vi "Log CAN Frame.vi"(8 "error in (no error)":errorcluster, 9 "timestamp":timestamp, 10 "CAN frame":T1 {"type" items=["CAN Data", "CAN Remote"]; "identifier" format="%.0x"}, 11 "tdms file":refnum<k34>) -> (0 "error out":errorcluster, 3 "tdms file out":refnum<k34>)   [LabVIEW 2014]
uses:
  <vilib>/RioEmbeddedCAN/RioEmbeddedCAN.llb/CANFrameControl.ctl
  MC/MC Temp 1.ctl
  MC/MC Temp 2.ctl
  MC/MC Temp 3.ctl
  MC/MC Position.ctl
  MC/MC Current.ctl
  MC/MC Voltage.ctl
  MC/MC State.ctl
  Inverter States.ctl
  Inverter Run Modes.ctl
  VSM States.ctl
  MC/MC Faults.ctl
  MC/MC Post Faults.ctl
  MC/MC Run Faults.ctl
  MC/MC Torque.ctl
  Global Data.vi
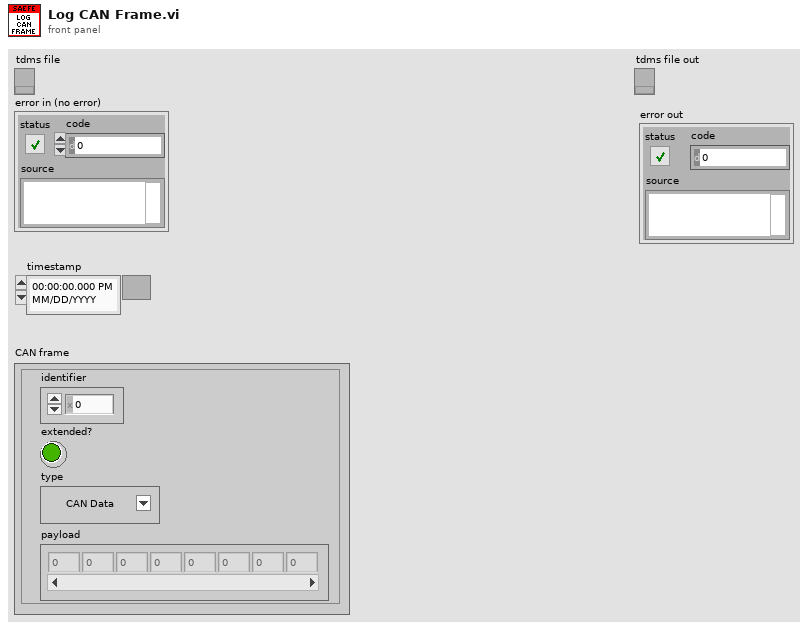
[diagram p1: front panel]
types:
  T1 = typedef "CANFrameControl.ctl" = cluster{"identifier":u32, "extended?":bool, "type":u8, "payload":u8[]}
  T2 = typedef "MC Temp 1.ctl" = cluster{"IGBT A (C)":dbl, "IGBT B (C)":dbl, "IGBT C (C)":dbl, "Gate Driver (C)":dbl}
  T3 = typedef "MC Temp 2.ctl" = cluster{"Control Board (C)":dbl, "RTD #1":dbl, "RTD #2":dbl, "RTD #3":dbl}
  T4 = typedef "MC Temp 3.ctl" = cluster{"RTD #4":dbl, "RTD #5":dbl, "Motor (C)":dbl, "T-Shudder":dbl}
  T5 = typedef "MC Position.ctl" = cluster{"Motor Angle":dbl, "Motor Speed":dbl, "Electrical Output Freq.":dbl, "Delta Resolver Filt.":dbl}
  T6 = typedef "MC Current.ctl" = cluster{"I-Phase A":dbl, "I-Phase B":dbl, "I-Phase C":dbl, "I-Battery":dbl}
  T7 = typedef "MC Voltage.ctl" = cluster{"V-Phase AB":dbl, "V-Phase BC":dbl, "V-Output":dbl, "V-Battery":dbl}
  T8 = typedef "MC State.ctl" = cluster{"Inverter":T9, "Inv. Run Mode":T10, "Inv. Command":enum16{"CAN Mode", "VSM Mode"}, "Inv. Enable":enum16{"Inverter Disabled", "Inverter Enabled"}, "Inv. Enable Lock":enum16{"Inverter Locked", "Inverter Unlocked"}, "Direction":enum16{"Forward", "Reverse/Stopped"}, "VSM States":T11, "Relay 1":bool, "Relay 2":bool, "Relay 3":bool, "Relay 4":bool}
  T9 = typedef "Inverter States.ctl" = enum16{"Power On", "Stop", "Open Loop", "Closed Loop", "Wait", "Internal", "Idle Run", "Idle Stop", ""}
  T10 = typedef "Inverter Run Modes.ctl" = enum16{"Torque Mode", "Speed Mode"}
  T11 = typedef "VSM States.ctl" = enum16{"VSM Start", "Pre-Charge Init", "Pre-Charge Active", "Pre-Charge Complete", "VSM Wait", "VSM Ready", "Motor Running", "Blink Fault Code", "Shutdown in Process", "Recycle Power"}
  T12 = typedef "MC Faults.ctl" = cluster{"POST":T13, "RUN":T14}
  T13 = typedef "MC Post Faults.ctl" = enum32{"None"}
  T14 = typedef "MC Run Faults.ctl" = enum32{"None"}
  T15 = typedef "MC Torque.ctl" = cluster{"T-Requested (Telem)":dbl, "T-Feedback":dbl}
  T16 = enum16{"Off", "On, Not Charging", "Charging", "Charging Finished", "Charging Error"}
  T17 = enum16{"Disconnected", "Pre-charging", "Main Charging", "Balancing", "Charging Finished OK", "Charging Error"}
  T18 = typedef "BMS Telemetry.ctl" = cluster{"Ignition":bool, "Charger Mains":bool, "Fast Charge":bool, "Simple Charger Enabled":bool, "Car State":enum16{"Off", "On, Not Charging", "Charging", "Charging Finished", "Charging Error"}, "Charging State":enum16{"Disconnected", "Pre-charging", "Main Charging", "Balancing", "Charging Finished OK", "Charging Error"}, "Charging Stage Duration":u16, "Last Charging Error":enum16{"No Error", "Cell Voltage Too Low", "No Comm from Cells so can't start", "Maximum charging stage duration expired", "No Comm from Cels so can't balande", "Cannot set balancing voltage", "Cell temps too high", "No Comms so can't determine temp", "# of Cells Mismatch", "Cells Overvoltage", "Cell Protection Event occured."}, "Number of Detected Cells":u8, "Under-Voltage":bool, "Over-Voltage":bool, "Overheat":bool, "Leakage":bool, "No Cell Comms":bool, "Low Voltage":bool, "High Temperature":bool, "Min Cell V":dbl, "Max Cell V":dbl, "Mean Cell V":dbl, "Total V":dbl, "Min Cell t":dbl, "Max Cell t":dbl, "Mean Cell t":dbl, "Cell-V's":dbl[], "Cell-t's":dbl[]}
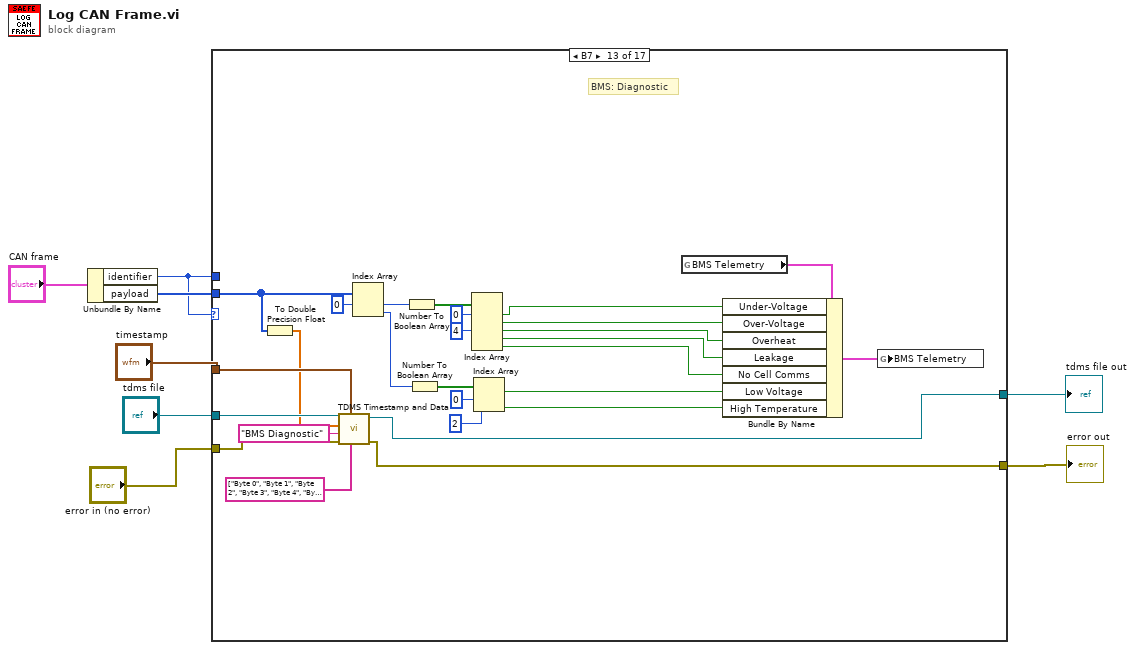
[diagram p0: block diagram]
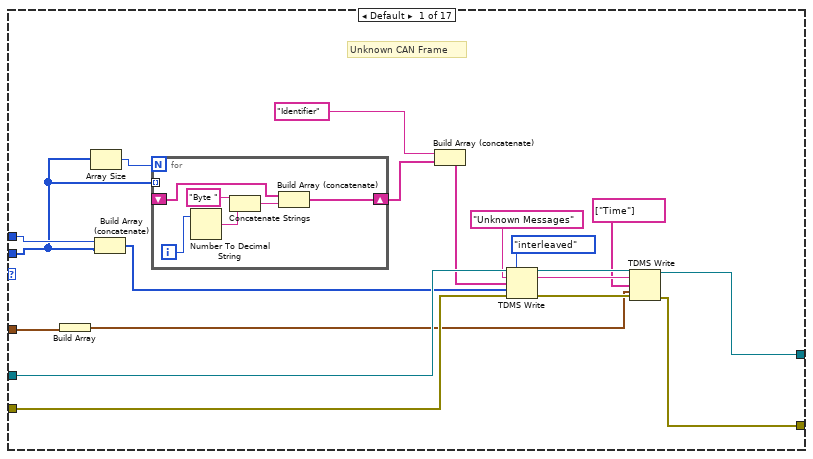
[diagram p2: hidden frame]
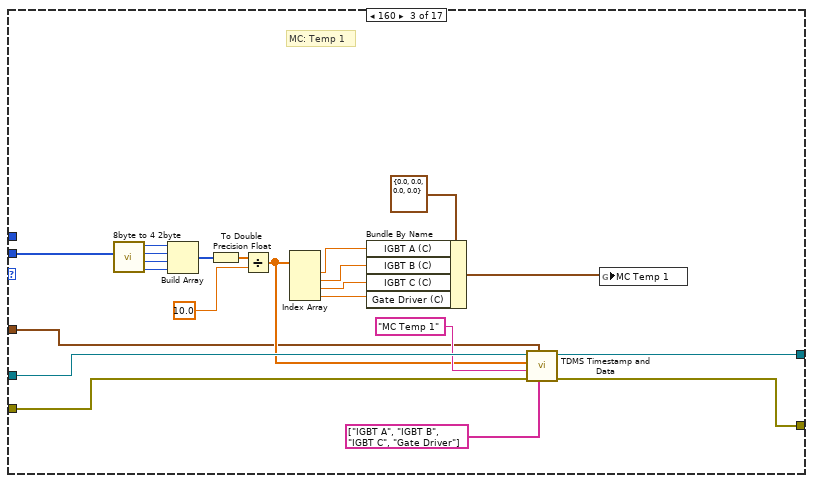
[diagram p4: hidden frame]
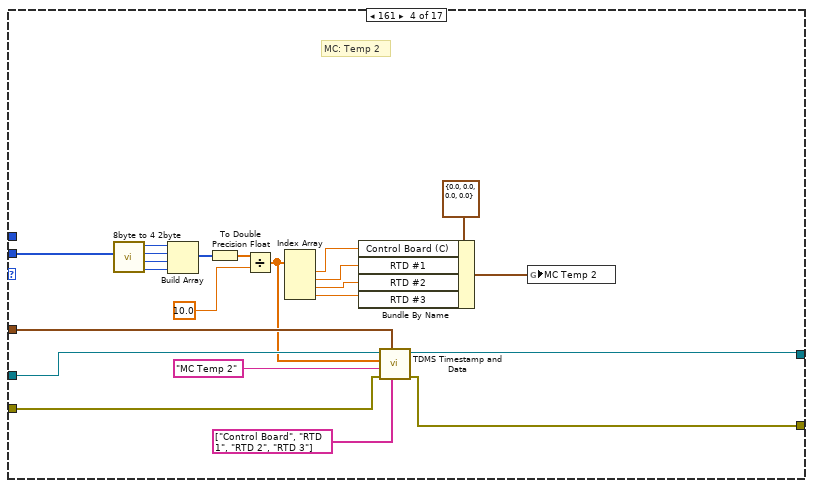
[diagram p5: hidden frame]
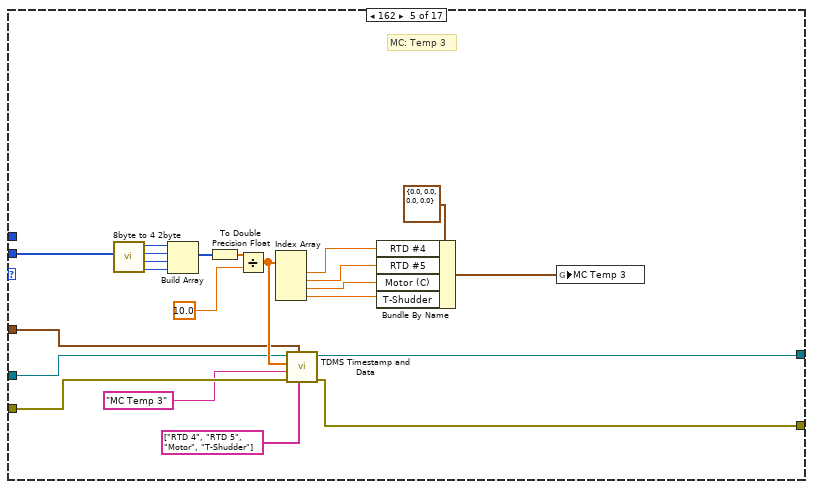
[diagram p6: hidden frame]
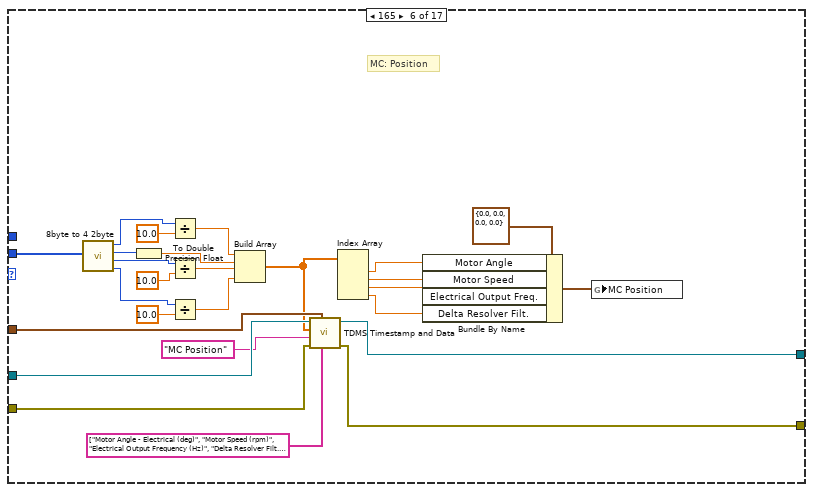
[diagram p7: hidden frame]
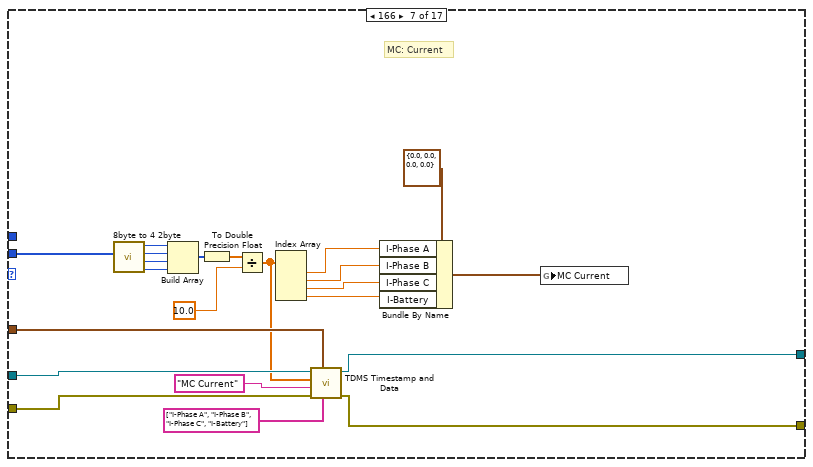
[diagram p8: hidden frame]
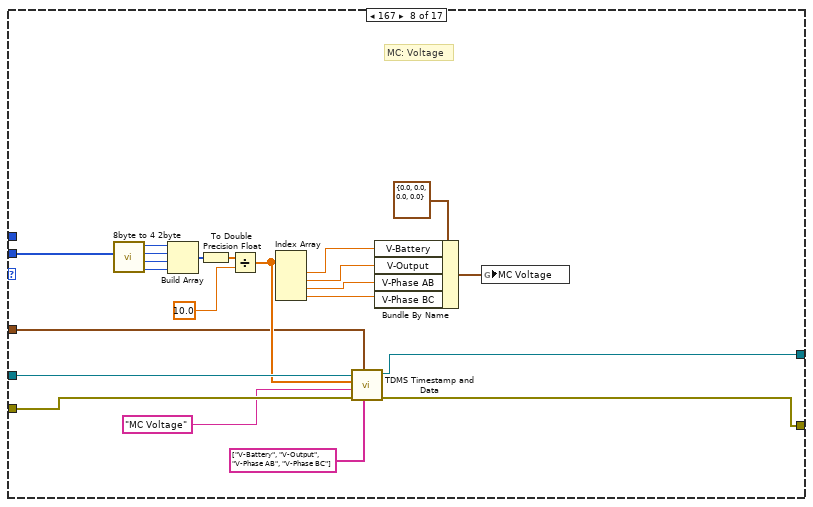
[diagram p9: hidden frame]
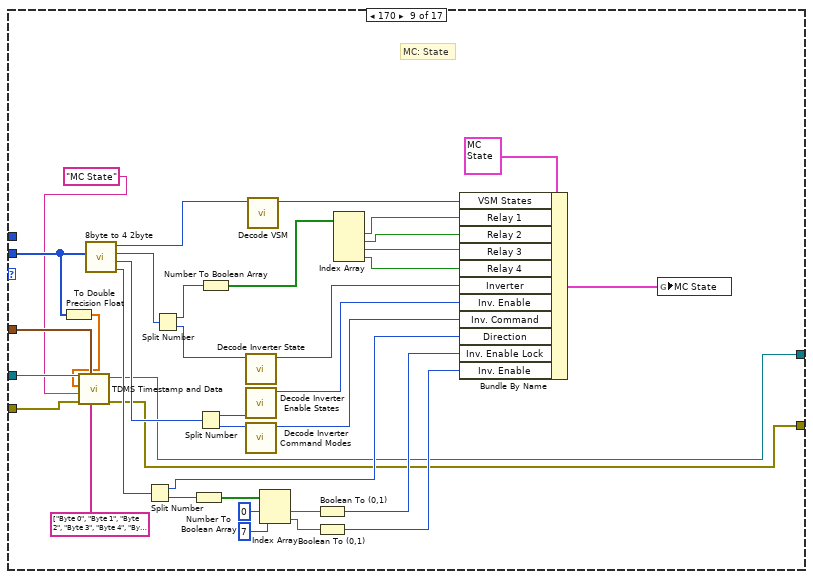
[diagram p10: hidden frame]
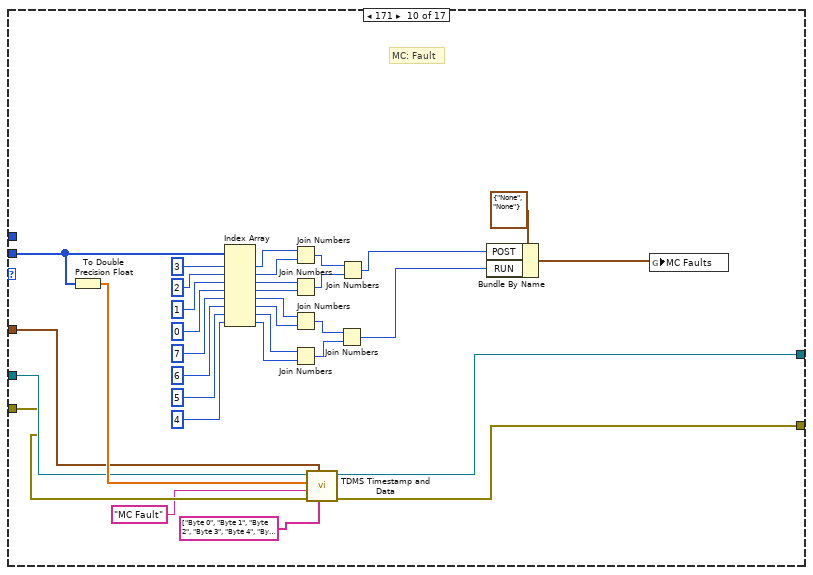
[diagram p11: hidden frame]
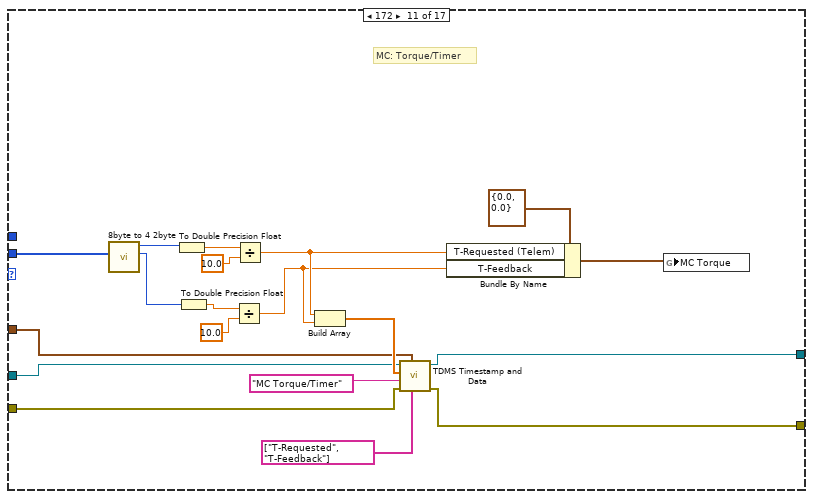
[diagram p12: hidden frame]
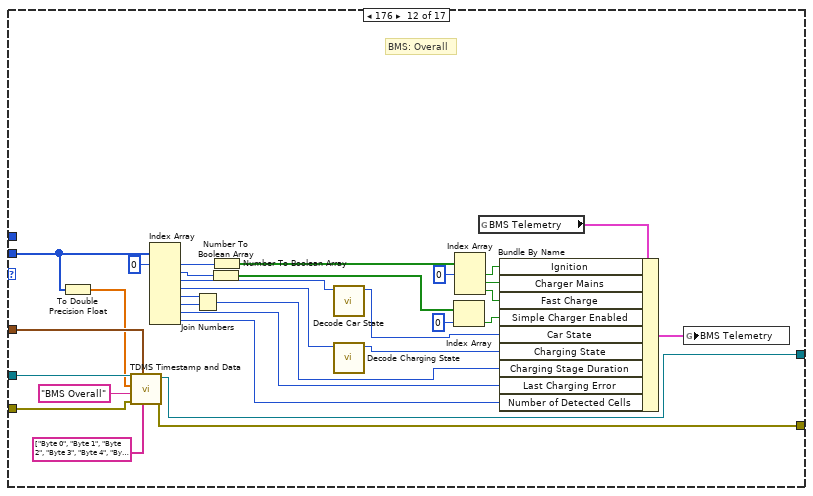
[diagram p13: hidden frame]
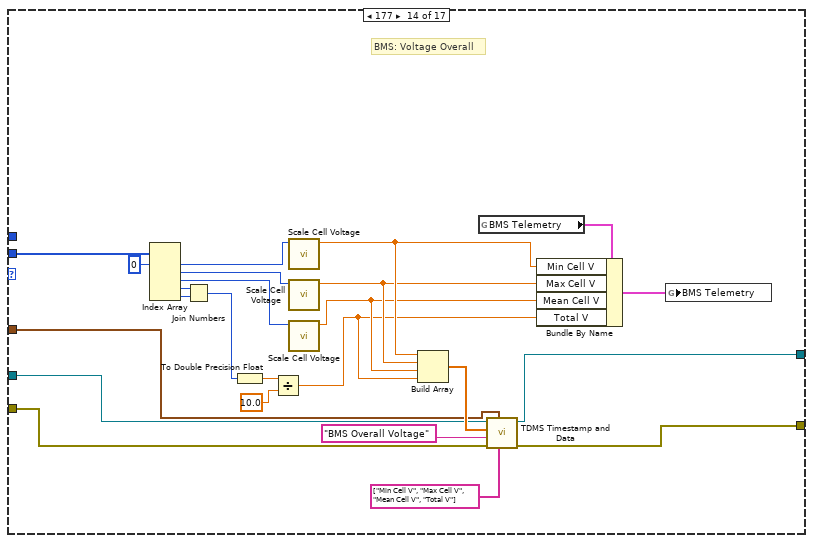
[diagram p14: hidden frame]
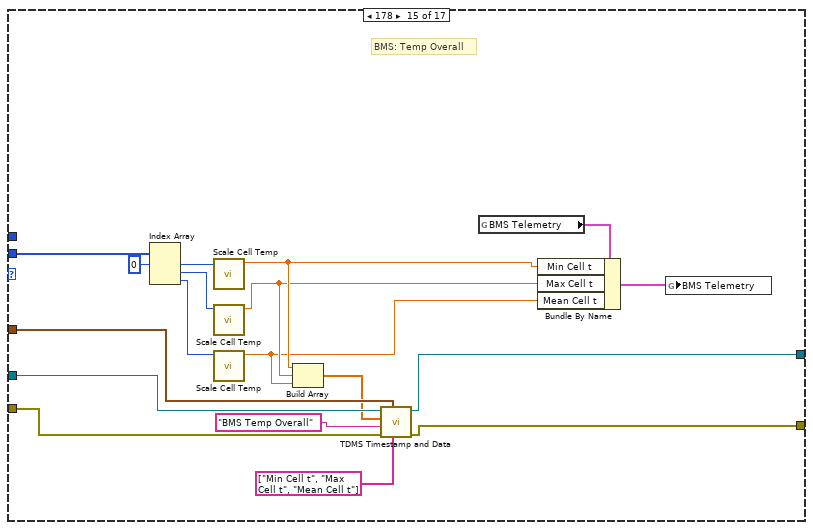
[diagram p15: hidden frame]
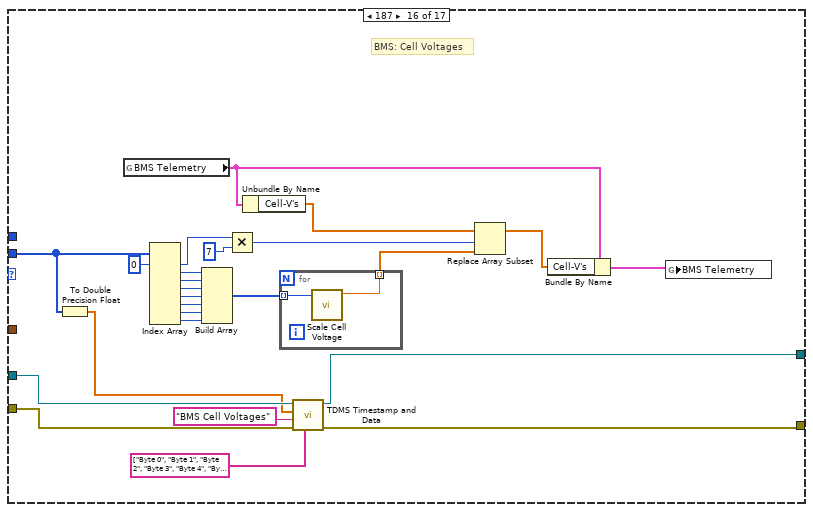
[diagram p16: hidden frame]
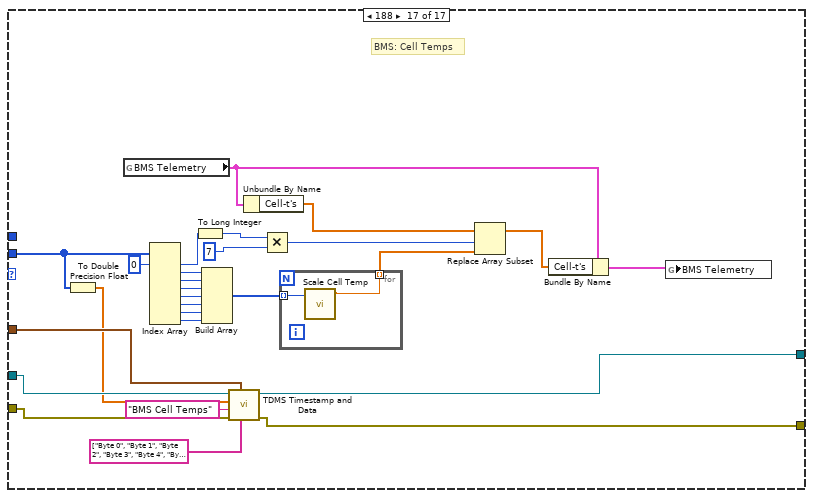
[diagram p17: hidden frame]
diagram:
  n1 = Unbundle By Name("CAN frame") -> ("identifier"=w5:u32, "payload"=w7:u8[])
  n2 = case shown="B7" w5 {
    tunnel: w5 -> [w27 _ _ _ _ _ _ _ _ _ _ _ _ _ _ _ _]
    tunnel: w7 -> [w9 _ w57 w79 w101 w127 w149 w171 w182 w219 w260 w266 w297 w340 w358 w362 w393]
    tunnel: "timestamp" -> [w14 _ w39 w67 w87 w115 w135 w156 w181 w216 w249 w267 w298 w323 w353 _ w398]
    tunnel: "tdms file" -> [w26 w35 w45 w66 w88 w114 w137 w159 w180 w217 w250 w269 w300 w325 w352 w368 w397]
    tunnel: [w11 w35 w42 w63 w85 w111 w131 w154 w177 w213 w246 w263 w294 w321 w344 w365 w394] -> w3
    tunnel: "error in (no error)" -> [w25 w34 w38 w65 w86 w113 w136 w158 w179 w215 w248 w268 w299 w324 w351 w367 w396]
    tunnel: [w12 w34 w41 w64 w84 w112 w130 w153 w176 w212 w245 w262 w293 w320 w343 w364 w395] -> w1
    frame Default {
      # "Unknown CAN Frame"
      n3 = Build Array(w14) -> (w13:timestamp[])
      n4 = Array Size(array=w9) -> (size(s)=w10:i32)
      n5 = Build Array (concatenate)(w27, w9) -> (w24:u32[])
      n6 = for {
        N: w10 -> [_]
        tunnel: w9 -> [_] mode=indexing
        shift-right: [w32] -> w23
        shift-left: _ -> [w28]
        i -> [w31]
        n7 = Number To Decimal String(number=w31) -> (decimal integer string=w30:string)  [unwired: 1 in]
        n8 = Concatenate Strings("Byte " ("string"), w30) -> (w33:string)
        n9 = Build Array (concatenate)(w28, w33) -> (w32:string[])
      }
      n10 = Build Array (concatenate)("Identifier", w23) -> (w21:string[])
      n11 = TDMS Write(0:w26, 1:enum16{"decimated", "interleaved"}."interleaved" ("data layout (0:decimated)"), 5:"Unknown Messages" ("group name in (Untitled)"), 7:w21, 9:w24, 11:w25) -> (4:w18:refnum<k34>, 6:w16:string, 15:w17:errorcluster)  [unwired: 1 out]
      n12 = TDMS Write(0:w18, 5:w16, 7:string[] ["Time"] ("channel name(s) in (Untitled)"), 9:w13, 11:w17) -> (4:w11:refnum<k34>, 15:w12:errorcluster)  [unwired: 1 in, 2 out]
    }
    frame 0 {
      # "Do nothing for NULL frame"
    }
    frame 160 {
      # "MC: Temp 1"
      n13 = call "8byte to 4 2byte.vi"("payload"=w57) -> ("7,6"=w53:i16, "5,4"=w54:i16, "3,2"=w55:i16, "1,0"=w56:i16)  [unwired: 7 in]
      n14 = Build Array(w56, w55, w54, w53) -> (w46:i16[])
      n15 = To Double Precision Float(number=w46) -> (double precision float=w47:dbl[])
      n16 = Divide(x=w47, y=10.0) -> (x/y=w40:dbl[])
      n17 = Index Array(array=w40) -> (element #1=w51:dbl, element #2=w50:dbl, element #3=w49:dbl, element #4=w48:dbl)  [unwired: 4 in]
      n18 = Bundle By Name(cluster=T2 {"IGBT A (C)"=0.0, "IGBT B (C)"=0.0, "IGBT C (C)"=0.0, "Gate Driver (C)"=0.0} ("MC Temp 1"), "IGBT A (C)"=w51, "IGBT B (C)"=w50, "IGBT C (C)"=w49, "Gate Driver (C)"=w48) -> (w36:T2)
      n19 = call "TDMS Timestamp and Data.vi"("channel name(s) in (Untitled)"=string[] ["IGBT A", "IGBT B", "IGBT C", "Gate Driver"], "timestamp"=w39, "error in (no error)"=w38, "group name in (Untitled)"="MC Temp 1", "Array"=w40, "Refnum in"=w45) -> ("error out"=w41:errorcluster, "Refnum out"=w42:refnum<k34>)  [unwired: 4 in]
      n20 = global write "Global Data.vi" "MC Temp 1"(w36) -> ()
    }
    frame 161 {
      # "MC: Temp 2"
      n21 = call "8byte to 4 2byte.vi"("payload"=w79) -> ("7,6"=w75:i16, "5,4"=w76:i16, "3,2"=w77:i16, "1,0"=w78:i16)  [unwired: 7 in]
      n22 = Build Array(w78, w77, w76, w75) -> (w68:i16[])
      n23 = To Double Precision Float(number=w68) -> (double precision float=w69:dbl[])
      n24 = Divide(x=w69, y=10.0) -> (x/y=w62:dbl[])
      n25 = Index Array(array=w62) -> (element #1=w73:dbl, element #2=w72:dbl, element #3=w71:dbl, element #4=w70:dbl)  [unwired: 4 in]
      n26 = Bundle By Name(cluster=T3 {"Control Board (C)"=0.0, "RTD #1"=0.0, "RTD #2"=0.0, "RTD #3"=0.0} ("MC Temp 2"), "Control Board (C)"=w73, "RTD #1"=w72, "RTD #2"=w71, "RTD #3"=w70) -> (w59:T3)
      n27 = call "TDMS Timestamp and Data.vi"("channel name(s) in (Untitled)"=string[] ["Control Board", "RTD 1", "RTD 2", "RTD 3"], "timestamp"=w67, "error in (no error)"=w65, "group name in (Untitled)"="MC Temp 2", "Array"=w62, "Refnum in"=w66) -> ("error out"=w64:errorcluster, "Refnum out"=w63:refnum<k34>)  [unwired: 4 in]
      n28 = global write "Global Data.vi" "MC Temp 2"(w59) -> ()
    }
    frame 162 {
      # "MC: Temp 3"
      n29 = call "8byte to 4 2byte.vi"("payload"=w101) -> ("7,6"=w97:i16, "5,4"=w98:i16, "3,2"=w99:i16, "1,0"=w100:i16)  [unwired: 7 in]
      n30 = Build Array(w100, w99, w98, w97) -> (w90:i16[])
      n31 = To Double Precision Float(number=w90) -> (double precision float=w91:dbl[])
      n32 = Divide(x=w91, y=10.0) -> (x/y=w89:dbl[])
      n33 = Index Array(array=w89) -> (element #1=w95:dbl, element #2=w94:dbl, element #3=w93:dbl, element #4=w92:dbl)  [unwired: 4 in]
      n34 = call "TDMS Timestamp and Data.vi"("channel name(s) in (Untitled)"=string[] ["RTD 4", "RTD 5", "Motor", "T-Shudder"], "timestamp"=w87, "error in (no error)"=w86, "group name in (Untitled)"="MC Temp 3", "Array"=w89, "Refnum in"=w88) -> ("error out"=w84:errorcluster, "Refnum out"=w85:refnum<k34>)  [unwired: 4 in]
      n35 = Bundle By Name(cluster=T4 {"RTD #4"=0.0, "RTD #5"=0.0, "Motor (C)"=0.0, "T-Shudder"=0.0} ("MC Temp 3"), "RTD #4"=w95, "RTD #5"=w94, "Motor (C)"=w93, "T-Shudder"=w92) -> (w81:T4)
      n36 = global write "Global Data.vi" "MC Temp 3"(w81) -> ()
    }
    frame 165 {
      # "MC: Position"
      n37 = call "8byte to 4 2byte.vi"("payload"=w127) -> ("7,6"=w122:i16, "5,4"=w123:i16, "3,2"=w117:i16, "1,0"=w126:i16)  [unwired: 7 in]
      n38 = To Double Precision Float(number=w117) -> (double precision float=w116:dbl)
      n39 = Divide(x=w126, y=10.0) -> (x/y=w121:dbl)
      n40 = Divide(x=w123, y=10.0) -> (x/y=w120:dbl)
      n41 = Divide(x=w122, y=10.0) -> (x/y=w119:dbl)
      n42 = Build Array(w121, w116, w120, w119) -> (w108:dbl[])
      n43 = call "TDMS Timestamp and Data.vi"("channel name(s) in (Untitled)"=string[] ["Motor Angle - Electrical (deg)", "Motor Speed (rpm)", "Electrical Output Frequency (Hz)", "Delta Resolver Filt. (deg)"], "timestamp"=w115, "error in (no error)"=w113, "group name in (Untitled)"="MC Position", "Array"=w108, "Refnum in"=w114) -> ("error out"=w112:errorcluster, "Refnum out"=w111:refnum<k34>)  [unwired: 4 in]
      n44 = Index Array(array=w108) -> (element #1=w107:dbl, element #2=w106:dbl, element #3=w105:dbl, element #4=w104:dbl)  [unwired: 4 in]
      n45 = Bundle By Name(cluster=T5 {"Motor Angle"=0.0, "Motor Speed"=0.0, "Electrical Output Freq."=0.0, "Delta Resolver Filt."=0.0} ("MC Position"), "Motor Angle"=w107, "Motor Speed"=w106, "Electrical Output Freq."=w105, "Delta Resolver Filt."=w104) -> (w102:T5)
      n46 = global write "Global Data.vi" "MC Position"(w102) -> ()
    }
    frame 166 {
      # "MC: Current"
      n47 = call "8byte to 4 2byte.vi"("payload"=w149) -> ("7,6"=w145:i16, "5,4"=w146:i16, "3,2"=w147:i16, "1,0"=w148:i16)  [unwired: 7 in]
      n48 = Build Array(w148, w147, w146, w145) -> (w138:i16[])
      n49 = To Double Precision Float(number=w138) -> (double precision float=w139:dbl[])
      n50 = Divide(x=w139, y=10.0) -> (x/y=w134:dbl[])
      n51 = Index Array(array=w134) -> (element #1=w143:dbl, element #2=w142:dbl, element #3=w141:dbl, element #4=w140:dbl)  [unwired: 4 in]
      n52 = call "TDMS Timestamp and Data.vi"("channel name(s) in (Untitled)"=string[] ["I-Phase A", "I-Phase B", "I-Phase C", "I-Battery"], "timestamp"=w135, "error in (no error)"=w136, "group name in (Untitled)"="MC Current", "Array"=w134, "Refnum in"=w137) -> ("error out"=w130:errorcluster, "Refnum out"=w131:refnum<k34>)  [unwired: 4 in]
      n53 = Bundle By Name(cluster=T6 {"I-Phase A"=0.0, "I-Phase B"=0.0, "I-Phase C"=0.0, "I-Battery"=0.0} ("MC Current"), "I-Phase A"=w143, "I-Phase B"=w142, "I-Phase C"=w141, "I-Battery"=w140) -> (w128:T6)
      n54 = global write "Global Data.vi" "MC Current"(w128) -> ()
    }
    frame 167 {
      # "MC: Voltage"
      n55 = call "8byte to 4 2byte.vi"("payload"=w171) -> ("7,6"=w167:i16, "5,4"=w168:i16, "3,2"=w169:i16, "1,0"=w170:i16)  [unwired: 7 in]
      n56 = Build Array(w170, w169, w168, w167) -> (w160:i16[])
      n57 = To Double Precision Float(number=w160) -> (double precision float=w161:dbl[])
      n58 = Divide(x=w161, y=10.0) -> (x/y=w157:dbl[])
      n59 = Index Array(array=w157) -> (element #1=w165:dbl, element #2=w164:dbl, element #3=w163:dbl, element #4=w162:dbl)  [unwired: 4 in]
      n60 = call "TDMS Timestamp and Data.vi"("channel name(s) in (Untitled)"=string[] ["V-Battery", "V-Output", "V-Phase AB", "V-Phase BC"], "timestamp"=w156, "error in (no error)"=w158, "group name in (Untitled)"="MC Voltage", "Array"=w157, "Refnum in"=w159) -> ("error out"=w153:errorcluster, "Refnum out"=w154:refnum<k34>)  [unwired: 4 in]
      n61 = Bundle By Name(cluster=T7 {"V-Phase AB"=0.0, "V-Phase BC"=0.0, "V-Output"=0.0, "V-Battery"=0.0} ("MC Voltage"), "V-Battery"=w165, "V-Output"=w164, "V-Phase AB"=w163, "V-Phase BC"=w162) -> (w150:T7)
      n62 = global write "Global Data.vi" "MC Voltage"(w150) -> ()
    }
    frame 170 {
      # "MC: State"
      n63 = To Double Precision Float(number=w182) -> (double precision float=w178:dbl[])
      n64 = call "TDMS Timestamp and Data.vi"("channel name(s) in (Untitled)"=string[] ["Byte 0", "Byte 1", "Byte 2", "Byte 3", "Byte 4", "Byte 5", "Byte 6", "Byte 7"], "timestamp"=w181, "error in (no error)"=w179, "group name in (Untitled)"="MC State", "Array"=w178, "Refnum in"=w180) -> ("error out"=w176:errorcluster, "Refnum out"=w177:refnum<k34>)  [unwired: 4 in]
      n65 = call "8byte to 4 2byte.vi"("payload"=w182) -> ("7,6"=w191:i16, "5,4"=w204:i16, "3,2"=w207:i16, "1,0"=w208:i16)  [unwired: 7 in]
      n66 = Split Number(x=w191) -> (hi(x)=w190:u8, lo(x)=w199:u8)
      n67 = Split Number(x=w207) -> (hi(x)=w183:u8, lo(x)=w206:u8)
      n68 = Number To Boolean Array(number=w199) -> (Boolean array=w198:bool[])
      n69 = Split Number(x=w204) -> (hi(x)=w203:u8, lo(x)=w201:u8)
      n70 = Number To Boolean Array(number=w183) -> (Boolean array=w189:bool[])
      n71 = call "Decode Inverter State.vi"("Byte In"=w206) -> ("Inverter State Out"=w205:T9)  [unwired: 10 in]
      n72 = call "Decode Inverter Enable States.vi"("Numeric"=w203) -> ("Inv. Enable"=w202:enum16{"Inverter Disabled", "Inverter Enabled"})  [unwired: 10 in]
      n73 = call "Decode Inverter Command Modes.vi"("Numeric"=w201) -> ("Inv. Command"=w200:enum16{"CAN Mode", "VSM Mode"})  [unwired: 10 in]
      n74 = call "Decode VSM.vi"("VSM Word"=w208) -> ("Enum"=w184:T11)  [unwired: 10 in]
      n75 = Index Array(array=w198, index #1=0 ("index"), index #2=7 ("index")) -> (element #1=w195:bool, element #2=w193:bool)
      n76 = Boolean To (0,1)(Boolean=w195) -> (0, 1=w194:i16)
      n77 = Boolean To (0,1)(Boolean=w193) -> (0, 1=w192:i16)
      n78 = Index Array(array=w189) -> (element #1=w188:bool, element #2=w187:bool, element #3=w186:bool, element #4=w185:bool)  [unwired: 4 in]
      n79 = Bundle By Name(cluster=T8 {"Inverter"=enum."Power On", "Inv. Run Mode"=enum."Torque Mode", "Inv. Command"=enum."CAN Mode", "Inv. Enable"=enum."Inverter Disabled", "Inv. Enable Lock"=enum."Inverter Locked", "Direction"=enum."Forward", "VSM States"=enum."VSM Start", "Relay 1"=FALSE, "Relay 2"=FALSE, "Relay 3"=FALSE, "Relay 4"=FALSE} ("MC State"), "VSM States"=w184, "Relay 1"=w188, "Relay 2"=w187, "Relay 3"=w186, "Relay 4"=w185, "Inverter"=w205, "Inv. Enable"=w202, "Inv. Command"=w200, "Direction"=w190, "Inv. Enable Lock"=w194, "Inv. Enable"=w192) -> (w172:T8)
      n80 = global write "Global Data.vi" "MC State"(w172) -> ()
    }
    frame 171 {
      # "MC: Fault"
      n81 = To Double Precision Float(number=w219) -> (double precision float=w218:dbl[])
      n82 = Index Array(array=w219, index #1=3 ("index"), index #2=2 ("index"), index #3=1 ("index"), index #4=0 ("index"), index #5=7 ("index"), index #6=6 ("index"), index #7=5 ("index"), index #8=4 ("index")) -> (element #1=w229:u8, element #2=w228:u8, element #3=w227:u8, element #4=w226:u8, element #5=w225:u8, element #6=w224:u8, element #7=w223:u8, element #8=w222:u8)
      n83 = Join Numbers(hi=w229, lo=w228) -> ((hi.lo)=w230:u16)
      n84 = Join Numbers(hi=w227, lo=w226) -> ((hi.lo)=w231:u16)
      n85 = Join Numbers(hi=w225, lo=w224) -> ((hi.lo)=w232:u16)
      n86 = Join Numbers(hi=w223, lo=w222) -> ((hi.lo)=w233:u16)
      n87 = call "TDMS Timestamp and Data.vi"("channel name(s) in (Untitled)"=string[] ["Byte 0", "Byte 1", "Byte 2", "Byte 3", "Byte 4", "Byte 5", "Byte 6", "Byte 7"], "timestamp"=w216, "error in (no error)"=w215, "group name in (Untitled)"="MC Fault", "Array"=w218, "Refnum in"=w217) -> ("error out"=w212:errorcluster, "Refnum out"=w213:refnum<k34>)  [unwired: 4 in]
      n88 = Join Numbers(hi=w232, lo=w233) -> ((hi.lo)=w220:u32)
      n89 = Join Numbers(hi=w230, lo=w231) -> ((hi.lo)=w221:u32)
      n90 = Bundle By Name(cluster=T12 {"POST"=enum."None", "RUN"=enum."None"} ("MC Faults"), "POST"=w221, "RUN"=w220) -> (w209:T12)
      n91 = global write "Global Data.vi" "MC Faults"(w209) -> ()
    }
    frame 172 {
      # "MC: Torque/Timer"
      n92 = call "8byte to 4 2byte.vi"("payload"=w260) -> ("3,2"=w256:i16, "1,0"=w259:i16)  [unwired: 7 in, 2 out]
      n93 = To Double Precision Float(number=w259) -> (double precision float=w258:dbl)
      n94 = To Double Precision Float(number=w256) -> (double precision float=w255:dbl)
      n95 = Divide(x=w255, y=10.0) -> (x/y=w252:dbl)
      n96 = Divide(x=w258, y=10.0) -> (x/y=w253:dbl)
      n97 = Build Array(w253, w252) -> (w251:dbl[])
      n98 = call "TDMS Timestamp and Data.vi"("channel name(s) in (Untitled)"=string[] ["T-Requested", "T-Feedback"], "timestamp"=w249, "error in (no error)"=w248, "group name in (Untitled)"="MC Torque/Timer", "Array"=w251, "Refnum in"=w250) -> ("error out"=w245:errorcluster, "Refnum out"=w246:refnum<k34>)  [unwired: 4 in]
      n99 = Bundle By Name(cluster=T15 {"T-Requested (Telem)"=0.0, "T-Feedback"=0.0} ("MC Torque"), "T-Requested (Telem)"=w253, "T-Feedback"=w252) -> (w243:T15)
      n100 = global write "Global Data.vi" "MC Torque"(w243) -> ()
    }
    frame 176 {
      # "BMS: Overall"
      n101 = To Double Precision Float(number=w266) -> (double precision float=w265:dbl[])
      n102 = call "TDMS Timestamp and Data.vi"("channel name(s) in (Untitled)"=string[] ["Byte 0", "Byte 1", "Byte 2", "Byte 3", "Byte 4", "Byte 5", "Byte 6", "Byte 7"], "timestamp"=w267, "error in (no error)"=w268, "group name in (Untitled)"="BMS Overall", "Array"=w265, "Refnum in"=w269) -> ("error out"=w262:errorcluster, "Refnum out"=w263:refnum<k34>)  [unwired: 4 in]
      n103 = Index Array(array=w266, index #1=0 ("index")) -> (element #1=w288:u8, element #2=w282:u8, element #3=w277:u8, element #4=w276:u8, element #5=w274:u8, element #6=w273:u8, element #7=w271:u8, element #8=w270:u8)  [unwired: 7 in]
      n104 = Join Numbers(hi=w274, lo=w273) -> ((hi.lo)=w272:u16)
      n105 = Number To Boolean Array(number=w282) -> (Boolean array=w280:bool[])
      n106 = Number To Boolean Array(number=w288) -> (Boolean array=w287:bool[])
      n107 = call "Decode Car State.vi"("Numeric"=w277) -> ("Car State"=w278:T16)  [unwired: 10 in]
      n108 = call "Decode Charging State.vi"("Numeric"=w276) -> ("Charging State"=w275:T17)  [unwired: 10 in]
      n109 = Index Array(array=w280, index=0) -> (element=w281:bool)
      n110 = Index Array(array=w287, index #1=0 ("index")) -> (element #1=w285:bool, element #2=w284:bool, element #3=w283:bool)  [unwired: 2 in]
      n111 = global read "Global Data.vi" "BMS Telemetry"() -> (w291:T18)
      n112 = Bundle By Name(cluster=w291, "Ignition"=w285, "Charger Mains"=w284, "Fast Charge"=w283, "Simple Charger Enabled"=w281, "Car State"=w278, "Charging State"=w275, "Charging Stage Duration"=w272, "Last Charging Error"=w271, "Number of Detected Cells"=w270) -> (w290:T18)
      n113 = global write "Global Data.vi" "BMS Telemetry"(w290) -> ()
    }
    frame 183 {
      # "BMS: Diagnostic"
      n114 = To Double Precision Float(number=w297) -> (double precision float=w296:dbl[])
      n115 = call "TDMS Timestamp and Data.vi"("channel name(s) in (Untitled)"=string[] ["Byte 0", "Byte 1", "Byte 2", "Byte 3", "Byte 4", "Byte 5", "Byte 6", "Byte 7"], "timestamp"=w298, "error in (no error)"=w299, "group name in (Untitled)"="BMS Diagnostic", "Array"=w296, "Refnum in"=w300) -> ("error out"=w293:errorcluster, "Refnum out"=w294:refnum<k34>)  [unwired: 4 in]
      n116 = Index Array(array=w297, index #1=0 ("index")) -> (element #1=w315:u8, element #2=w306:u8)  [unwired: 1 in]
      n117 = Number To Boolean Array(number=w315) -> (Boolean array=w314:bool[])
      n118 = Number To Boolean Array(number=w306) -> (Boolean array=w305:bool[])
      n119 = Index Array(array=w314, index #1=0 ("index"), index #3=4 ("index")) -> (element #1=w312:bool, element #2=w311:bool, element #3=w309:bool, element #4=w308:bool, element #5=w307:bool)  [unwired: 3 in]
      n120 = Index Array(array=w305, index #1=0 ("index"), index #2=2 ("index")) -> (element #1=w302:bool, element #2=w301:bool)
      n121 = global read "Global Data.vi" "BMS Telemetry"() -> (w318:T18)
      n122 = Bundle By Name(cluster=w318, "Under-Voltage"=w312, "Over-Voltage"=w311, "Overheat"=w309, "Leakage"=w308, "No Cell Comms"=w307, "Low Voltage"=w302, "High Temperature"=w301) -> (w317:T18)
      n123 = global write "Global Data.vi" "BMS Telemetry"(w317) -> ()
    }
    frame 177 {
      # "BMS: Voltage Overall"
      n124 = Index Array(array=w340, index #1=0 ("index")) -> (element #1=w338:u8, element #2=w337:u8, element #3=w336:u8, element #4=w335:u8, element #5=w334:u8)  [unwired: 4 in]
      n125 = Join Numbers(hi=w335, lo=w334) -> ((hi.lo)=w333:u16)
      n126 = To Double Precision Float(number=w333) -> (double precision float=w332:dbl)
      n127 = Divide(x=w332, y=10.0) -> (x/y=w327:dbl)
      n128 = call "Scale Cell Voltage.vi"("Numeric in"=w338) -> ("Numeric out"=w330:dbl)  [unwired: 10 in]
      n129 = call "Scale Cell Voltage.vi"("Numeric in"=w337) -> ("Numeric out"=w329:dbl)  [unwired: 10 in]
      n130 = call "Scale Cell Voltage.vi"("Numeric in"=w336) -> ("Numeric out"=w328:dbl)  [unwired: 10 in]
      n131 = Build Array(w330, w329, w328, w327) -> (w326:dbl[])
      n132 = global read "Global Data.vi" "BMS Telemetry"() -> (w342:T18)
      n133 = call "TDMS Timestamp and Data.vi"("channel name(s) in (Untitled)"=string[] ["Min Cell V", "Max Cell V", "Mean Cell V", "Total V"], "timestamp"=w323, "error in (no error)"=w324, "group name in (Untitled)"="BMS Overall Voltage", "Array"=w326, "Refnum in"=w325) -> ("error out"=w320:errorcluster, "Refnum out"=w321:refnum<k34>)  [unwired: 4 in]
      n134 = Bundle By Name(cluster=w342, "Min Cell V"=w330, "Max Cell V"=w329, "Mean Cell V"=w328, "Total V"=w327) -> (w341:T18)
      n135 = global write "Global Data.vi" "BMS Telemetry"(w341) -> ()
    }
    frame 178 {
      # "BMS: Temp Overall"
      n136 = Index Array(array=w358, index #1=0 ("index")) -> (element #1=w356:u8, element #2=w355:u8, element #3=w354:u8)  [unwired: 2 in]
      n137 = call "Scale Cell Temp.vi"("Numeric in"=w356) -> ("Numeric out"=w350:dbl)  [unwired: 10 in]
      n138 = call "Scale Cell Temp.vi"("Numeric in"=w355) -> ("Numeric out"=w349:dbl)  [unwired: 10 in]
      n139 = call "Scale Cell Temp.vi"("Numeric in"=w354) -> ("Numeric out"=w348:dbl)  [unwired: 10 in]
      n140 = Build Array(w350, w349, w348) -> (w347:dbl[])
      n141 = call "TDMS Timestamp and Data.vi"("channel name(s) in (Untitled)"=string[] ["Min Cell t", "Max Cell t", "Mean Cell t"], "timestamp"=w353, "error in (no error)"=w351, "group name in (Untitled)"="BMS Temp Overall", "Array"=w347, "Refnum in"=w352) -> ("error out"=w343:errorcluster, "Refnum out"=w344:refnum<k34>)  [unwired: 4 in]
      n142 = global read "Global Data.vi" "BMS Telemetry"() -> (w360:T18)
      n143 = Bundle By Name(cluster=w360, "Min Cell t"=w350, "Max Cell t"=w349, "Mean Cell t"=w348) -> (w359:T18)
      n144 = global write "Global Data.vi" "BMS Telemetry"(w359) -> ()
    }
    frame 187 {
      # "BMS: Cell Voltages"
      n145 = To Double Precision Float(number=w362) -> (double precision float=w361:dbl[])
      n146 = global read "Global Data.vi" "BMS Telemetry"() -> (w381:T18)
      n147 = Index Array(array=w362, index #1=0 ("index")) -> (element #1=w383:u8, element #2=w378:u8, element #3=w377:u8, element #4=w376:u8, element #5=w375:u8, element #6=w374:u8, element #7=w373:u8, element #8=w372:u8)  [unwired: 7 in]
      n148 = Build Array(w378, w377, w376, w375, w374, w373, w372) -> (w371:u8[])
      n149 = Multiply(x=w383, y=7) -> (x*y=w369:i32)
      n150 = Unbundle By Name(w381) -> ("Cell-V's"=w380:dbl[])
      n151 = for {
        tunnel: w371 -> [w387] mode=indexing
        tunnel: [w386] -> w370 mode=indexing
        n152 = call "Scale Cell Voltage.vi"("Numeric in"=w387) -> ("Numeric out"=w386:dbl)  [unwired: 10 in]
      }
      n153 = call "TDMS Timestamp and Data.vi"("channel name(s) in (Untitled)"=string[] ["Byte 0", "Byte 1", "Byte 2", "Byte 3", "Byte 4", "Byte 5", "Byte 6", "Byte 7"], "error in (no error)"=w367, "group name in (Untitled)"="BMS Cell Voltages", "Array"=w361, "Refnum in"=w368) -> ("error out"=w364:errorcluster, "Refnum out"=w365:refnum<k34>)  [unwired: 5 in]
      n154 = Replace Array Subset(array=w380, new element=w370, index=w369) -> (w379:dbl[])
      n155 = Bundle By Name(cluster=w381, "Cell-V's"=w379) -> (w385:T18)
      n156 = global write "Global Data.vi" "BMS Telemetry"(w385) -> ()
    }
    frame 188 {
      # "BMS: Cell Temps"
      n157 = To Double Precision Float(number=w393) -> (double precision float=w392:dbl[])
      n158 = global read "Global Data.vi" "BMS Telemetry"() -> (w411:T18)
      n159 = Index Array(array=w393, index #1=0 ("index")) -> (element #1=w388:u8, element #2=w408:u8, element #3=w407:u8, element #4=w406:u8, element #5=w405:u8, element #6=w404:u8, element #7=w403:u8, element #8=w402:u8)  [unwired: 7 in]
      n160 = To Long Integer(number=w388) -> (32bit integer=w389:i32)
      n161 = Build Array(w408, w407, w406, w405, w404, w403, w402) -> (w401:u8[])
      n162 = call "TDMS Timestamp and Data.vi"("channel name(s) in (Untitled)"=string[] ["Byte 0", "Byte 1", "Byte 2", "Byte 3", "Byte 4", "Byte 5", "Byte 6", "Byte 7"], "timestamp"=w398, "error in (no error)"=w396, "group name in (Untitled)"="BMS Cell Temps", "Array"=w392, "Refnum in"=w397) -> ("error out"=w395:errorcluster, "Refnum out"=w394:refnum<k34>)  [unwired: 4 in]
      n163 = Unbundle By Name(w411) -> ("Cell-t's"=w410:dbl[])
      n164 = Multiply(x=w389, y=7) -> (x*y=w399:i32)
      n165 = for {
        tunnel: w401 -> [w415] mode=indexing
        tunnel: [w416] -> w400 mode=indexing
        n166 = call "Scale Cell Temp.vi"("Numeric in"=w415) -> ("Numeric out"=w416:dbl)  [unwired: 10 in]
      }
      n167 = Replace Array Subset(array=w410, new element=w400, index=w399) -> (w409:dbl[])
      n168 = Bundle By Name(cluster=w411, "Cell-t's"=w409) -> (w414:T18)
      n169 = global write "Global Data.vi" "BMS Telemetry"(w414) -> ()
    }
  }
  "tdms file out" <- w3
  "error out" <- w1
